vi "fn Get Servers.vi"(8 "error in (no error)":errorcluster, 11 "address (localhost)":string) -> (0 "error out":errorcluster, 3 "[Servers]":string[](array[string]))   [LabVIEW 2024, in "LV_OPC.lvlib"]
doc: "LVOPC_API int fnGetServers(char* address, char* buf[]);"
uses:
  LV_OPC.lvlib
  LVOPC64.dll
panel:
  out "list out":string
  out "address out":string
  out "function return":i32
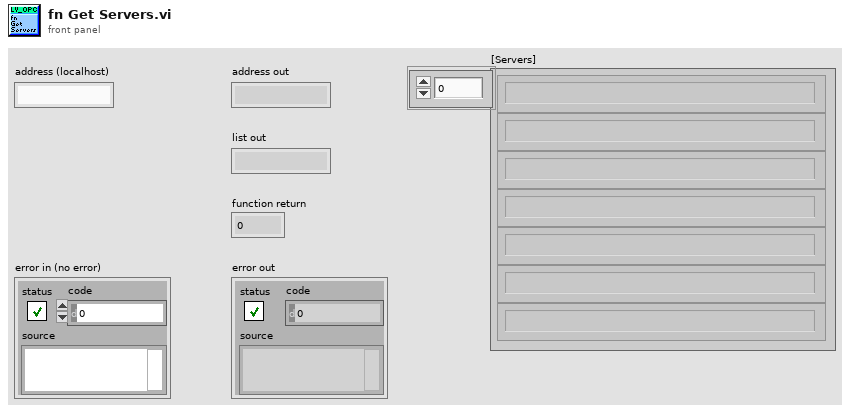
[diagram p1: front panel]
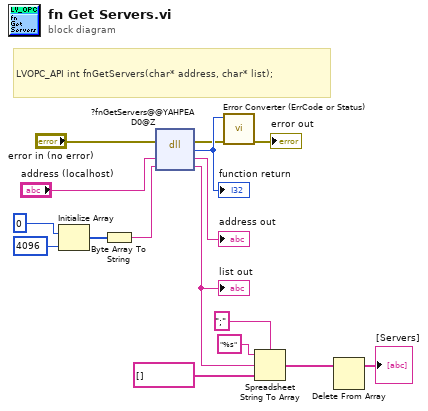
[diagram p0: block diagram]
diagram:
  # "LVOPC_API int fnGetServers(char* address, char* list);"
  n1 = Initialize Array(u8 0 ("element"), 4096 ("dimension size")) -> (w9:u8[])
  n2 = Byte Array To String(unsigned byte array=w9) -> (string=w8:string)
  n3 = dll-call lib="C:/Users/Andrey/Desktop/LV_OPC-Client-x64/LV_OPC_Test/OPC.DLL/LVOPC64.*" fn="?fnGetServers@@YAHPEAD0@Z"(error in="error in (no error)", "address"="address (localhost)", "list"=w8) -> (error out=w13:errorcluster, "return type"=w16:i32, "address"=→"address out":string, "list"=w3:string)  [unwired: 2 in, 1 out]
  "function return" <- w16
  "list out" <- w3
  n4 = call "Error Converter (ErrCode or Status).vi"("error in (no error)"=w13, "error code"=w16) -> ("error out"=→"error out":errorcluster)  [unwired: 9 in]
  n5 = Spreadsheet String To Array(delimiter (Tab)=";", format string="%s", spreadsheet string=w3, array type (2D Dbl)=string[] []) -> (array=w2:string[])
  n6 = Delete From Array(array=w2) -> (array with subset deleted=→"[Servers]":string[])  [unwired: 2 in, 1 out]
